vi "getLeftData_ShootDualTalonSRX.vi"() -> (0 "Raw encoder counts  L":dbl, 1 "Applied Output  L":dbl format="%.5f", 2 "Encoder Velocity Units Per 100ms L":dbl format="%.5f", 3 "Target Velocity Units per 100ms L":dbl format="%.5f", 4 "Distance FT L":dbl format="%.5f", 5 "Speed  FT/SEC L":dbl format="%.5f", 7 "Speed Dmd  FT/SEC L":dbl format="%.5f")   [LabVIEW 2019, in "ShootDualTalonSRX_Motor_Pair.lvlib"]
uses:
  ShootDualTalonSRX_Motor_Pair.lvlib
  globals_ShootDualTalonSRX.vi
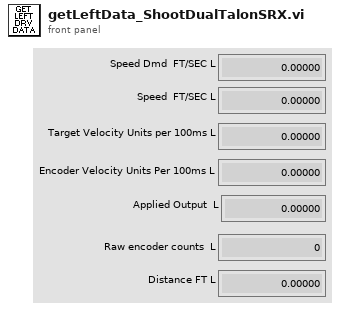
[diagram p1: front panel]
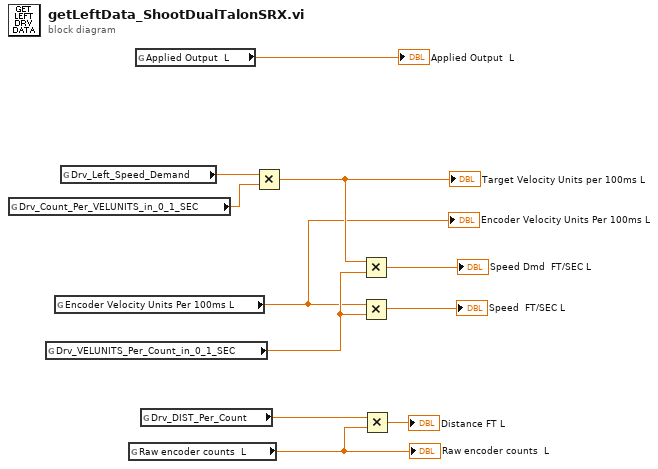
[diagram p0: block diagram]
diagram:
  n1 = global read "globals_ShootDualTalonSRX.vi" "Drv_Count_Per_VELUNITS_in_0_1_SEC"() -> (w7:dbl)
  n2 = global read "globals_ShootDualTalonSRX.vi" "Drv_VELUNITS_Per_Count_in_0_1_SEC"() -> (w5:dbl)
  n3 = global read "globals_ShootDualTalonSRX.vi" "Encoder Velocity Units Per 100ms L"() -> (w2:dbl)
  "Encoder Velocity Units Per 100ms L" <- w2
  n4 = global read "globals_ShootDualTalonSRX.vi" "Drv_Left_Speed_Demand"() -> (w4:dbl)
  n5 = global read "globals_ShootDualTalonSRX.vi" "Raw encoder counts  L"() -> (w3:dbl)
  "Raw encoder counts  L" <- w3
  n6 = global read "globals_ShootDualTalonSRX.vi" "Applied Output  L"() -> (→"Applied Output  L":dbl)
  n7 = global read "globals_ShootDualTalonSRX.vi" "Drv_DIST_Per_Count"() -> (w6:dbl)
  n8 = Multiply(x=w4, y=w7) -> (x*y=w9:dbl)
  "Target Velocity Units per 100ms L" <- w9
  n9 = Multiply(x=w9, y=w5) -> (x*y=→"Speed Dmd  FT/SEC L":dbl)
  n10 = Multiply(x=w2, y=w5) -> (x*y=→"Speed  FT/SEC L":dbl)
  n11 = Multiply(x=w6, y=w3) -> (x*y=→"Distance FT L":dbl)
